vi "limit_switch.vi"(8 "error in (no error)":errorcluster caption="エラー入力（エラーなし）", 10 "Velocity (1000)":u16=1000 max=5000 step=1, 11 "VISAリソース名":refnum<visa-resource-name>) -> (0 "error out":errorcluster caption="エラー出力", 3 "VISAリソース名（出力）":refnum<visa-resource-name>)   [LabVIEW 2017]
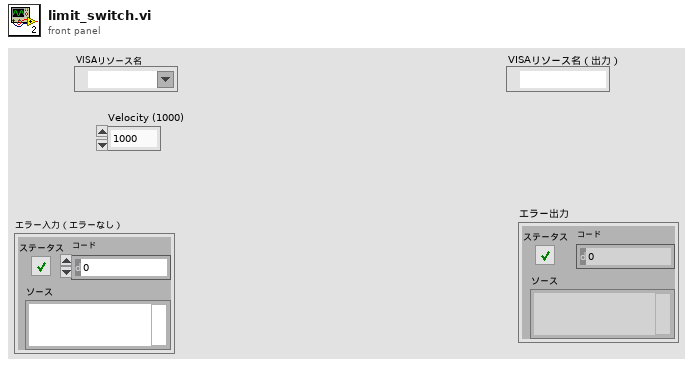
[diagram p1: front panel]
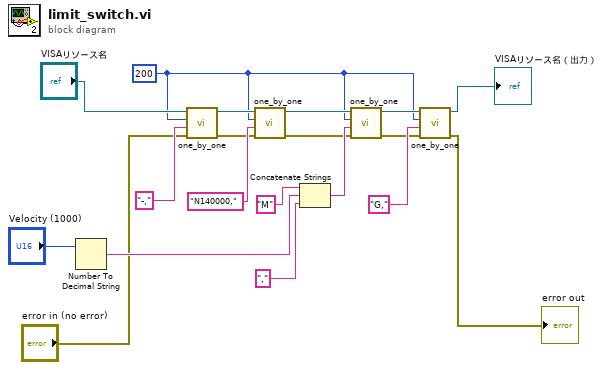
[diagram p0: block diagram]
diagram:
  w3 = 200
  n1 = Number To Decimal String(number="Velocity (1000)") -> (decimal integer string=w12:string)  [unwired: 1 in]
  n2 = call "one_by_one.vi"("error in (no error)"="error in (no error)", "入力文字"="-,", "待機 (200ms)"=w3, "VISAリソース名"="VISAリソース名") -> ("error out"=w8:errorcluster, "VISAリソース名出力"=w16:refnum<visa-resource-name>)  [unwired: 6 in]
  n3 = call "one_by_one.vi"("error in (no error)"=w8, "入力文字"="N140000,", "待機 (200ms)"=w3, "VISAリソース名"=w16) -> ("error out"=w7:errorcluster, "VISAリソース名出力"=w15:refnum<visa-resource-name>)  [unwired: 6 in]
  n4 = Concatenate Strings("M", w12, ",") -> (w10:string)
  n5 = call "one_by_one.vi"("error in (no error)"=w7, "入力文字"=w10, "待機 (200ms)"=w3, "VISAリソース名"=w15) -> ("error out"=w5:errorcluster, "VISAリソース名出力"=w4:refnum<visa-resource-name>)  [unwired: 6 in]
  n6 = call "one_by_one.vi"("error in (no error)"=w5, "入力文字"="G,", "待機 (200ms)"=w3, "VISAリソース名"=w4) -> ("error out"=→"error out":errorcluster, "VISAリソース名出力"=→"VISAリソース名（出力）":refnum<visa-resource-name>)  [unwired: 6 in]
